vi "Config Global.vi"() -> ()   [LabVIEW 2016, in "Log4Lv.lvlib"]
uses:
  Log4Lv.lvlib
panel:
  out "Config":T1={"LogName"="", "Level"=enum."Info", "LogFolder"=path "", "MaxFileSize"=0, "FileExtension"="", "TimeSytle"="", "LogStyle"=""}
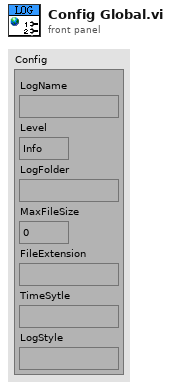
[diagram p1: front panel]
types:
  T1 = cluster{"LogName":string, "Level":enum16{"Disable", "Error", "Warn", "Info", "Debug"}, "LogFolder":path, "MaxFileSize":i32, "FileExtension":string, "TimeSytle":string, "LogStyle":string}
diagram:
